vi "Test MQTT-3.8.4-3.vi"(8 "error in (no error)":errorcluster) -> (0 "error out":errorcluster)   [LabVIEW 2013]
uses:
  source/Control Packets/SUBSCRIBE/Topic Subscription -- cluster.ctl
  source/Control Packets/ControlPacket/QualityOfService -- enum.ctl
  source/Client/Client.lvclass
  <vilib>/addons/_JKI Toolkits/Caraya/classes/Test/Test.lvclass
  source/Control Packets/ControlPacket/ControlPacket.lvclass
  source/Control Packets/SUBSCRIBE/SUBSCRIBE.lvclass
  source/MQTT_Base/MQTT_Base.lvclass
  <vilib>/addons/_JKI Toolkits/Caraya/classes/Assert/Assert.lvclass
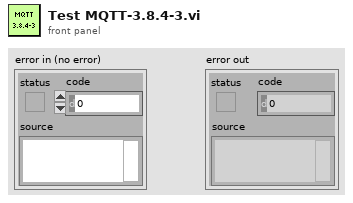
[diagram p1: front panel]
types:
  T1 = typedef "SUBSCRIBE.lvclass/Topic Subscription -- cluster.ctl" = cluster{"Topic Filter":string, "QoS":T2}
  T2 = typedef "ControlPacket.lvclass/QualityOfService -- enum.ctl" = enum16{"0 (At Most Once)", "1 (At Least Once)", "2 (Exactly Once)"}
  T3 = typedef "SUBACK.lvclass/Subscription Success Code.ctl" = cluster{"Subscription Failure":bool, "QoS":T2}
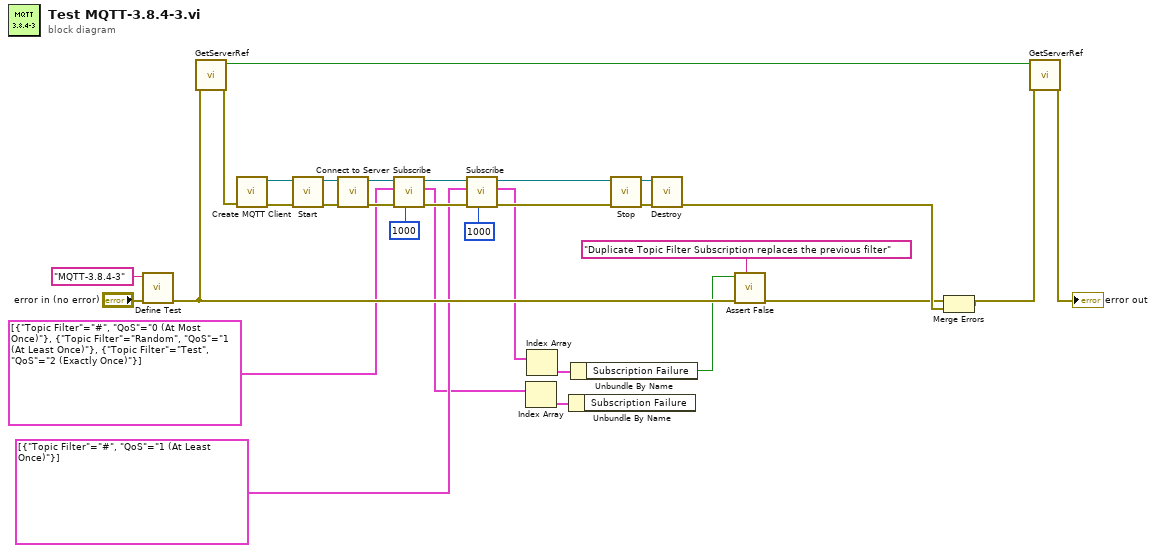
[diagram p0: block diagram]
diagram:
  n1 = call <vilib>:"Define Test.vi"("error in (no error)"="error in (no error)", "Label (VI Title)"="MQTT-3.8.4-3") -> ("error out"=w15:errorcluster)  [unwired: 9 in]
  n2 = call "GetServerRef.vi"("error in"=w15) -> ("error out"=w28:errorcluster, "Created"=w29:bool)  [unwired: 8 in, 1 out]
  n3 = call "Create MQTT Client.vi"("error in (no error)"=w28) -> ("error out"=w17:errorcluster, "Client out"=w18:refnum<class "Client.lvclass">)  [unwired: 9 in]
  n4 = call "Start.vi"("error in (no error)"=w17, "MQTT_Base in"=w18) -> ("error out"=w24:errorcluster, "MQTT_Base out"=w25:refnum<class "Client.lvclass">)  [unwired: 7 in, 1 out]
  n5 = call "Connect to Server.vi"("error in (no error)"=w24, "Client in"=w25) -> ("error out"=w20:errorcluster, "Client out"=w21:refnum<class "Client.lvclass">)  [unwired: 7 in, 1 out]
  n6 = call "Subscribe.vi"("timeout (1000 ms)"=1000, "error in (no error)"=w20, "Topic Subscriptions"=T1[] [{"Topic Filter"="#", "QoS"=enum."0 (At Most Once)"}, {"Topic Filter"="Random", "QoS"=enum."1 (At Least Once)"}, {"Topic Filter"="Test", "QoS"=enum."2 (Exactly Once)"}], "MQTT_Base in"=w21) -> ("error out"=w9:errorcluster, "Subscription Success"=w5:T3[], "MQTT_Base out"=w11:refnum<class "Client.lvclass">)  [unwired: 4 in, 1 out]
  n7 = call "Subscribe.vi"("timeout (1000 ms)"=1000, "error in (no error)"=w9, "Topic Subscriptions"=T1[] [{"Topic Filter"="#", "QoS"=enum."1 (At Least Once)"}], "MQTT_Base in"=w11) -> ("error out"=w8:errorcluster, "Subscription Success"=w4:T3[], "MQTT_Base out"=w10:refnum<class "Client.lvclass">)  [unwired: 4 in, 1 out]
  n8 = Index Array(array=w5) -> (element=w2:T3)  [unwired: 1 in]
  n9 = Index Array(array=w4) -> (element=w3:T3)  [unwired: 1 in]
  n10 = Unbundle By Name(w2) -> ()  [unwired: 1 out]
  n11 = Unbundle By Name(w3) -> ("Subscription Failure"=w1:bool)
  n12 = call "Stop.vi"("error in (no error)"=w8, "MQTT_Base in"=w10) -> ("error out"=w22:errorcluster, "MQTT_Base out"=w23:refnum<class "Client.lvclass">)  [unwired: 7 in, 1 out]
  n13 = call-dynamic "Destroy.vi"("error in (no error)"=w22, "Client in"=w23) -> ("error out"=w14:errorcluster)  [unwired: 8 in, 1 out]
  n14 = call <vilib>:"Assert False.vi"("Label"="Duplicate Topic Filter Subscription replaces the previous filter", "error in (no error)"=w15, "False?"=w1) -> ("error out"=w13:errorcluster)  [unwired: 8 in]
  n15 = Merge Errors(w13, w14) -> (w16:errorcluster)
  n16 = call "GetServerRef.vi"("error in"=w16, "Destroy (F)"=w29) -> ("error out"=→"error out":errorcluster)  [unwired: 7 in, 2 out]
